vi "Ramp up motors.vi"(6 "Last BR motor value":dbl, 8 "Last BL motor value":dbl, 9 "Last FR motor value":dbl, 10 "Set motor value":dbl, 11 "Last FL motor value":dbl) -> (0 "Next FR motor value":dbl, 1 "Next BR motor value":dbl, 2 "Next BL motor value":dbl, 3 "Next FL motor value":dbl)   [LabVIEW 2013]
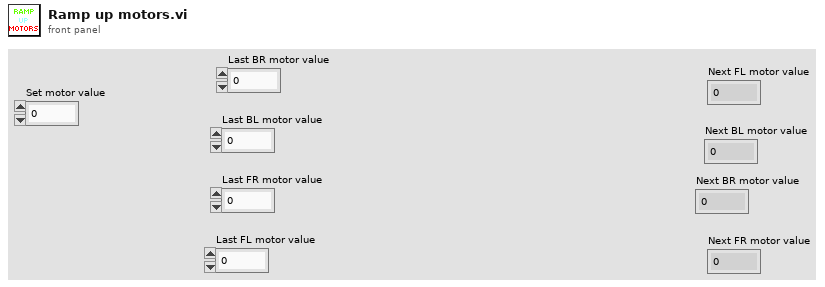
[diagram p1: front panel]
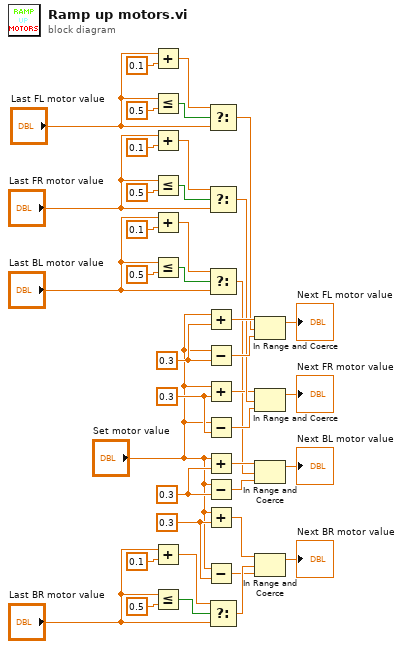
[diagram p0: block diagram]
diagram:
  w3 = 0.3
  w20 = 0.3
  w23 = 0.3
  w40 = 0.3
  n1 = Add(x="Last FL motor value", y=0.1) -> (x+y=w41:dbl)
  n2 = Less Or Equal?(x="Last FL motor value", y=0.5) -> (x <= y?=w34:bool)
  n3 = Add(x="Last FR motor value", y=0.1) -> (x+y=w22:dbl)
  n4 = Less Or Equal?(x="Last FR motor value", y=0.5) -> (x <= y?=w29:bool)
  n5 = Add(x="Last BL motor value", y=0.1) -> (x+y=w21:dbl)
  n6 = Less Or Equal?(x="Last BL motor value", y=0.5) -> (x <= y?=w14:bool)
  n7 = Add(x="Last BR motor value", y=0.1) -> (x+y=w2:dbl)
  n8 = Less Or Equal?(x="Last BR motor value", y=0.5) -> (x <= y?=w9:bool)
  n9 = Add(x="Set motor value", y=w40) -> (x+y=w38:dbl)
  n10 = Subtract(x="Set motor value", y=w40) -> (x-y=w39:dbl)
  n11 = Add(x="Set motor value", y=w23) -> (x+y=w25:dbl)
  n12 = Subtract(x="Set motor value", y=w23) -> (x-y=w24:dbl)
  n13 = Add(x="Set motor value", y=w20) -> (x+y=w18:dbl)
  n14 = Subtract(x="Set motor value", y=w20) -> (x-y=w19:dbl)
  n15 = Add(x="Set motor value", y=w3) -> (x+y=w5:dbl)
  n16 = Subtract(x="Set motor value", y=w3) -> (x-y=w4:dbl)
  n17 = Select(t=w41, s=w34, f="Last FL motor value") -> (s? t:f=w36:dbl)
  n18 = Select(t=w22, s=w29, f="Last FR motor value") -> (s? t:f=w27:dbl)
  n19 = Select(t=w21, s=w14, f="Last BL motor value") -> (s? t:f=w16:dbl)
  n20 = Select(t=w2, s=w9, f="Last BR motor value") -> (s? t:f=w7:dbl)
  n21 = In Range and Coerce(upper limit=w38, x=w36, lower limit=w39) -> (coerced(x)=→"Next FL motor value":dbl)  [unwired: 1 out]
  n22 = In Range and Coerce(upper limit=w25, x=w27, lower limit=w24) -> (coerced(x)=→"Next FR motor value":dbl)  [unwired: 1 out]
  n23 = In Range and Coerce(upper limit=w18, x=w16, lower limit=w19) -> (coerced(x)=→"Next BL motor value":dbl)  [unwired: 1 out]
  n24 = In Range and Coerce(upper limit=w5, x=w7, lower limit=w4) -> (coerced(x)=→"Next BR motor value":dbl)  [unwired: 1 out]
